vi "OnlyKeepCircularDepedentItems.vi"(11 "LibraryDependency In":map{path, T1}(c390)) -> (3 "LibraryDependency Out":map{path, T1}(c390))   [LabVIEW 2020, in "DependencyChecker.lvlib"]
uses:
  DependencyChecker.lvlib
  LibraryDependentInfo.vi
  <vilib>/Utility/lvfile.llb/FT_FileTypes.ctl
  <vilib>/Utility/lvfile.llb/NI_FileType.lvlib
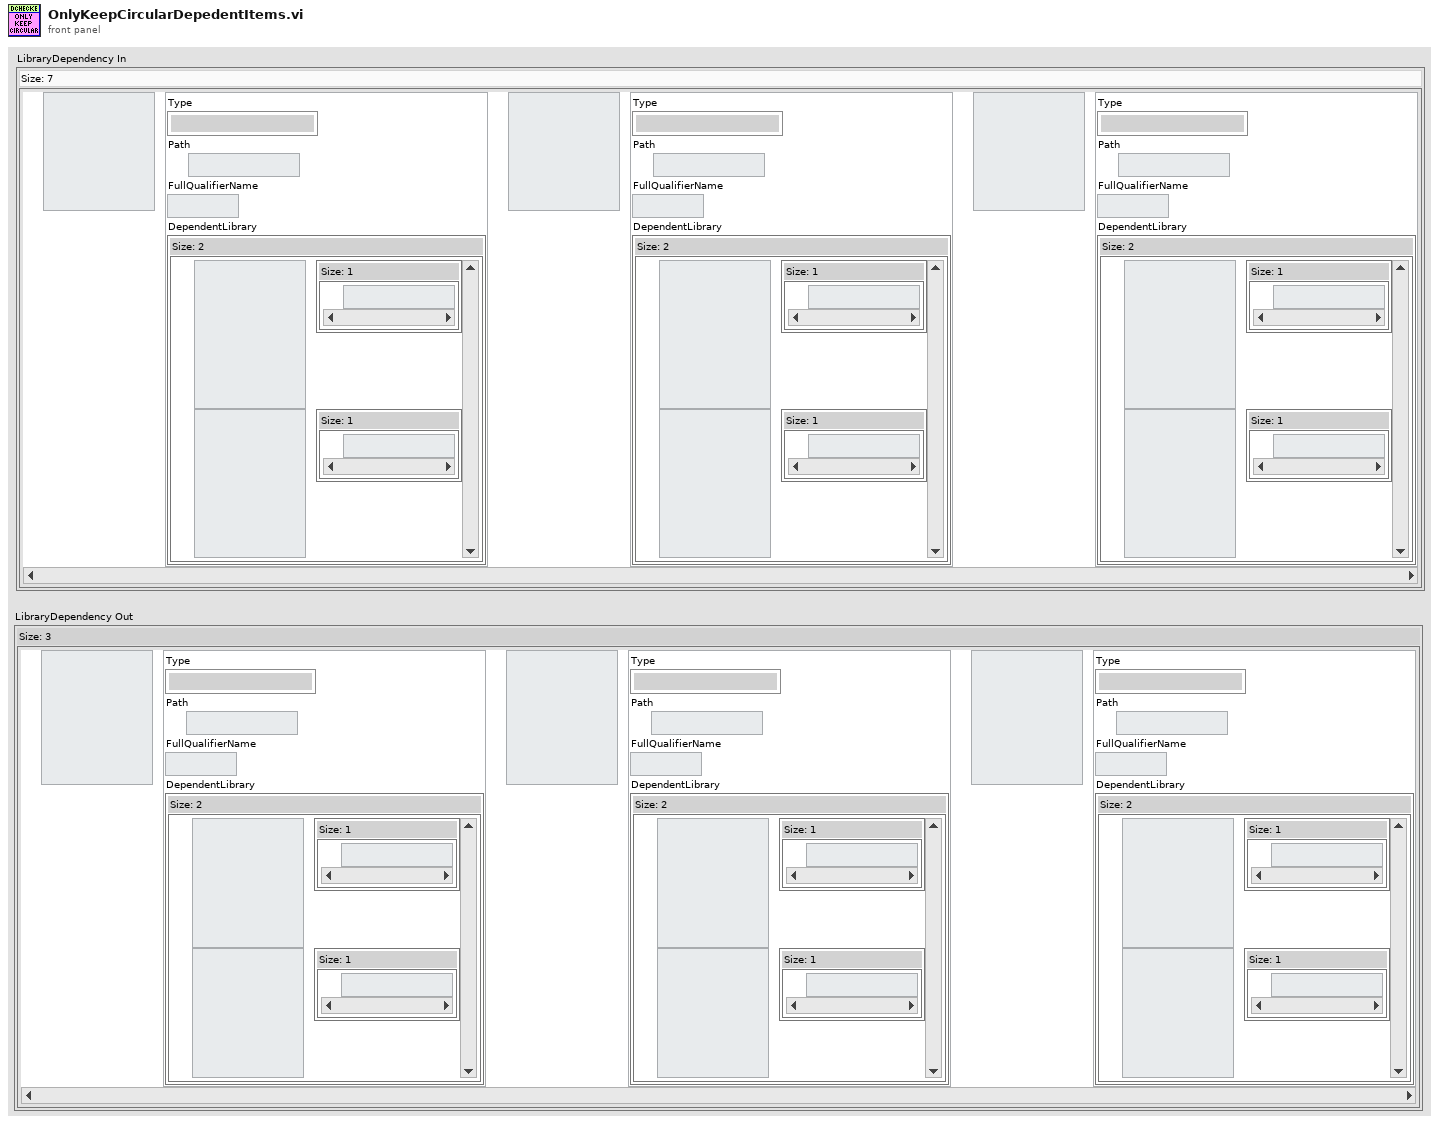
[diagram p1: front panel]
types:
  T1 = typedef "DependencyChecker.lvlib/LibraryDependentInfo.vi" = cluster{"Type":T2, "Path":path, "FullQualifierName":string, "DependentLibrary":map{path, set{path}}}
  T2 = typedef "NI_FileType.lvlib/FT_FileTypes.ctl" = enum32{"Invalid file/path", "Unknown type", "Instrument", "Control", "Polymorphic VI", "Project", "Library", "LVClass", "XControl", "XNode", "CIN", "Run-time menu", "Palette menu", "LLB", "Shortcut", "Directory", "Class Private Data Control", "Statechart", "MathScript .m file", "Ladder Diagram", "LVLibp"}
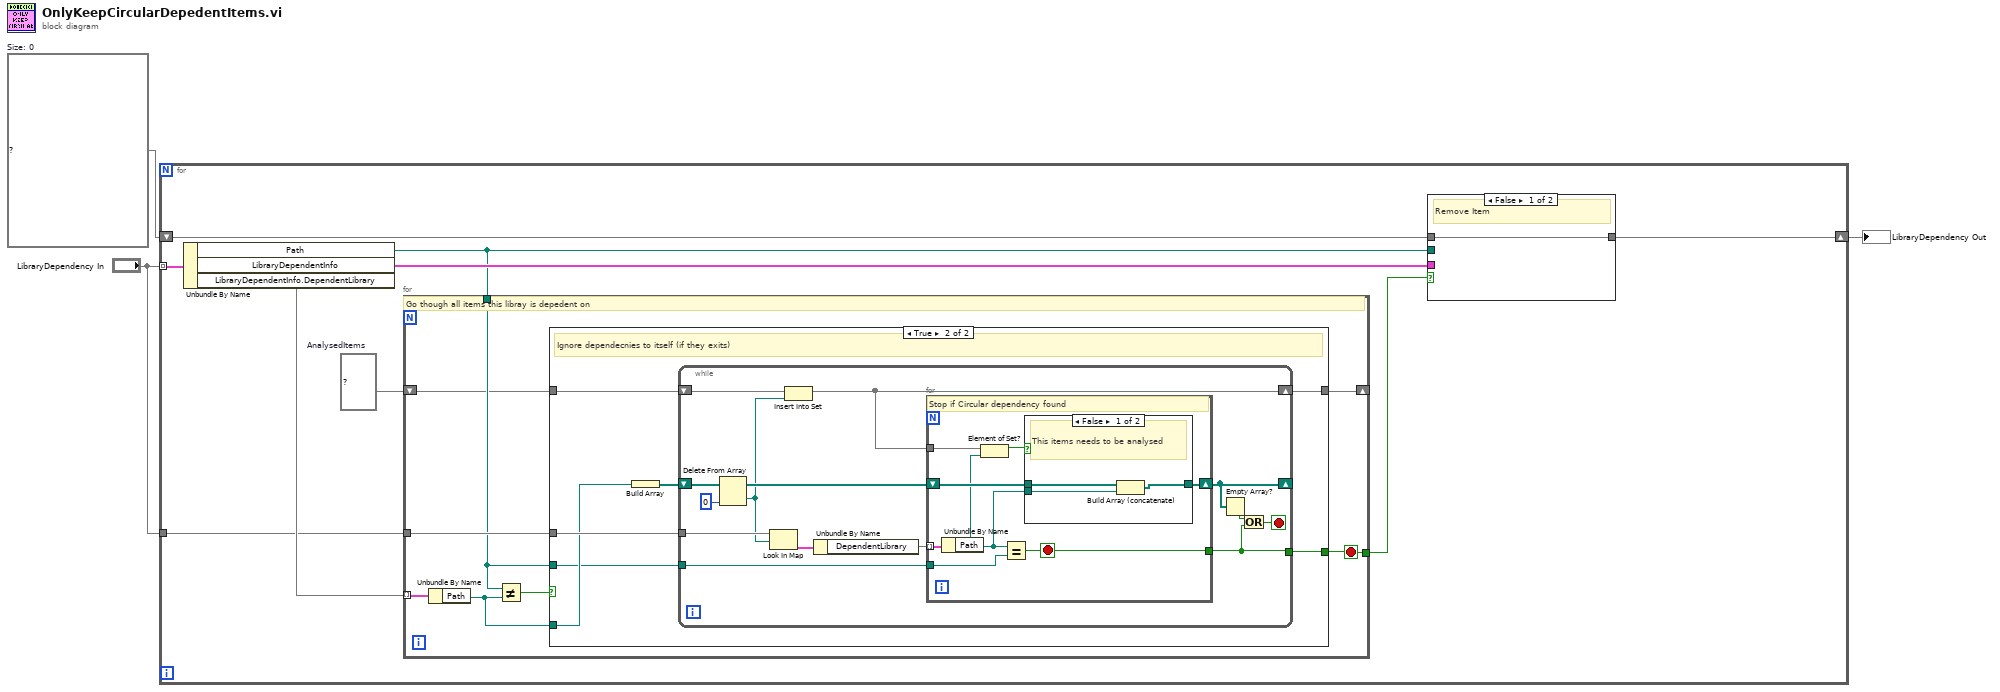
[diagram p0: block diagram]
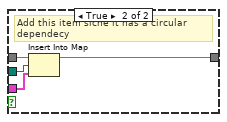
[diagram p4: hidden frame]
diagram:
  w2 = map{path, T1} {}  # Size: 0
  n1 = for {
    tunnel: "LibraryDependency In" -> [w12] mode=indexing
    shift-right: [w11] -> w3
    shift-left: w2 -> [w7]
    tunnel: "LibraryDependency In" -> [w4]
    w5 = set{path} {}  # AnalysedItems
    n2 = Unbundle By Name(w12) -> ("Path"=w8:path, "LibraryDependentInfo"=w10:T1, "LibraryDependentInfo.DependentLibrary"=w9:map{path, set{path}})
    n3 = for {
      tunnel: w9 -> [w20] mode=indexing
      tunnel: w8 -> [w16]
      tunnel: w4 -> [w18]
      tunnel: [w15] -> w6
      shift-right: [w13] -> _
      shift-left: w5 -> [w14]
      stop <- w15 stop-if-true
      # "Go though all items this libray is depedent on"
      n4 = Unbundle By Name(w20) -> ("Path"=w17:path)
      n5 = Not Equal?(x=w16, y=w17) -> (x != y?=w19:bool)
      n6 = case shown="True" w19 {
        tunnel: w18 -> [_ w28]
        tunnel: w17 -> [_ w27]
        tunnel: w16 -> [_ w25]
        tunnel: [_ w24] -> w15
        tunnel: w14 -> [w21 w23]
        tunnel: [w21 w22] -> w13
        frame False {
          # "Ignore Self depedency (if exists)"
        }
        frame True {
          # "Ignore dependecnies to itself (if they exits)"
          n7 = Build Array(w27) -> (w26:path[])
          n8 = while {
            tunnel: w28 -> [w42]
            shift-right: [w32] -> _
            shift-left: w26 -> [w39]
            tunnel: w25 -> [w37]
            tunnel: [w30] -> w24
            shift-right: [w33] -> w22
            shift-left: w23 -> [w35]
            stop <- w29 stop-if-true
            n9 = Delete From Array(array=w39, index=0) -> (deleted portion=w34:path, array with subset deleted=w36:path[])  [unwired: 1 in]
            n10 = Look In Map(map=w42, key=w34) -> (value=w41:T1)  [unwired: 1 in, 1 out]
            n11 = Insert Into Set(10:w34, 11:w35) -> (3:w33:set{path})  [unwired: 1 out]
            n12 = Unbundle By Name(w41) -> ("DependentLibrary"=w40:map{path, set{path}})
            n13 = for {
              tunnel: w40 -> [w50] mode=indexing
              tunnel: w37 -> [w49]
              tunnel: [w48] -> w30
              shift-right: [w44] -> w32
              shift-left: w36 -> [w45]
              tunnel: w33 -> [w47]
              stop <- w48 stop-if-true
              # "Stop if Circular dependency found"
              n14 = Unbundle By Name(w50) -> ("Path"=w43:path)
              n15 = Element of Set?(10:w43, 11:w47) -> (3:w46:bool)
              n16 = Equal?(x=w43, y=w49) -> (x = y?=w48:bool)
              n17 = case shown="False" w46 {
                tunnel: w45 -> [w53 w54]
                tunnel: [w52 w54] -> w44
                tunnel: w43 -> [w51 _]
                frame False {
                  # "This items needs to be analysed"
                  n18 = Build Array (concatenate)(w53, w51) -> (w52:path[])
                }
                frame True {
                  # "This item has already been analysed"
                }
              }
            }
            n19 = Empty Array?(array=w32) -> (empty?=w31:bool)
            n20 = Or(x=w31, y=w30) -> (x .or. y?=w29:bool)
          }
        }
      }
    }
    n21 = case shown="False" w6 {
      tunnel: w7 -> [w55 w59]
      tunnel: w8 -> [_ w57]
      tunnel: [w55 w58] -> w11
      tunnel: w10 -> [_ w56]
      frame False {
        # "Remove Item"
      }
      frame True {
        # "Add this item sicne it has a circular dependecy"
        n22 = Insert Into Map(map in=w59, key=w57, value=w56) -> (map out=w58:map{path, T1})  [unwired: 2 out]
      }
    }
  }
  "LibraryDependency Out" <- w3
